vi "LVPortInvokeMethod.vi"(7 "Result Type or Value to update (if any)":variant, 9 "Arguments (if nameless array then multi arguments)":variant, 10 "Method Name":string, 11 "pID":string) -> (0 "Method Executed ?":bool, 2 "Has Result ?":bool, 3 "Result (if any)":variant)   [LabVIEW 2017]
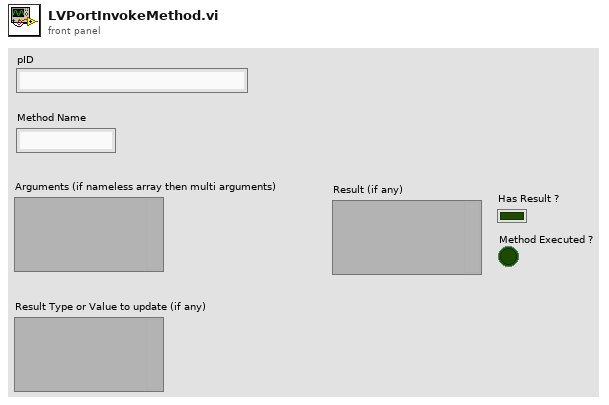
[diagram p1: front panel]
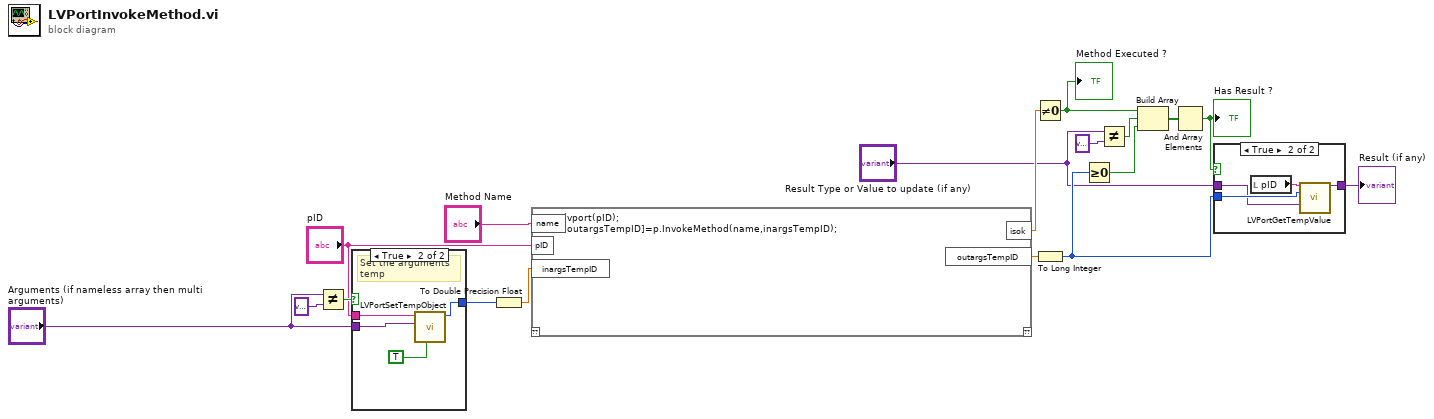
[diagram p0: block diagram]
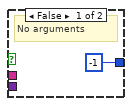
[diagram p3: hidden frame]
diagram:
  n1 = Not Equal?(x="Arguments (if nameless array then multi arguments)", y=variant) -> (x != y?=w18:bool)
  n2 = case shown="True" w18 {
    tunnel: "pID" -> [_ w23]
    tunnel: "Arguments (if nameless array then multi arguments)" -> [_ w22]
    tunnel: [-1 ("ID (Validated)") w21] -> w15
    frame False {
      # "No arguments"
    }
    frame True {
      # "Set the arguments temp"
      n3 = call "LVPortSetTempObject.vi"("Nameless Array as Object"=TRUE, "Value"=w22, "pID"=w23) -> ("ID (Validated)"=w21:i32)  [unwired: 6 in, 2 out]
    }
  }
  n4 = To Double Precision Float(number=w15) -> (double precision float=w14:dbl)
  n5 = script code="p=mlvport(pID);\n[isok,outargsTempID]=p.InvokeMethod(name,inargsTempID);"("pID"="pID", "inargsTempID"=w14, "name"="Method Name") -> ("isok"=w11:dbl, "outargsTempID"=w7:dbl)  [unwired: 1 in, 1 out]
  n6 = Not Equal To 0?(x=w11) -> (x != 0?=w9:bool)
  "Method Executed ?" <- w9
  n7 = To Long Integer(number=w7) -> (32bit integer=w4:i32)
  n8 = Greater Or Equal To 0?(x=w4) -> (x >= 0?=w6:bool)
  n9 = Not Equal?(x="Result Type or Value to update (if any)", y=variant) -> (x != y?=w8:bool)
  n10 = Build Array(w9, w8, w6) -> (w10:bool[])
  n11 = And Array Elements(Boolean array=w10) -> (logical AND=w1:bool)
  "Has Result ?" <- w1
  n12 = case shown="True" w1 {
    tunnel: w4 -> [_ w27]
    tunnel: "Result Type or Value to update (if any)" -> [w24 w26]
    tunnel: [w24 w25] -> w2
    frame False {
    }
    frame True {
      n13 = local read "pID"() -> (w28:string)
      n14 = call "LVPortGetTempValue.vi"("pID"=w28, "Object ID"=w27, "Value Type (Or value to update)"=w26) -> ("Value"=w25:variant)  [unwired: 11 in, 1 out]
    }
  }
  "Result (if any)" <- w2
